vi "bool-cmd-test.vi"() -> ()   [LabVIEW 2019]
uses:
  <vilib>/Rock Robotics/WPI/ThirdParty/JAS_Junk/TrajLib/VI/BoolCmd_Recv_Internal.vi
  <vilib>/Rock Robotics/WPI/ThirdParty/JAS_Junk/TrajLib/VI/BoolCmd_Send_Internal.vi
  <vilib>/Rock Robotics/WPI/ThirdParty/JAS_Junk/TrajLib/VI/BoolCmd_ObtainQueue.vi
  <vilib>/Rock Robotics/WPI/ThirdParty/JAS_Junk/TrajLib/Trajectory_Library.lvlib
panel:
  out "Two Falling Edge":bool
  out "error out 8":errorcluster
  out "error out 7":errorcluster
  out "Two":bool
  out "One Always":bool
  out "One Edge":bool
  out "error out 6":errorcluster
  out "error out 5":errorcluster
  out "error out 4":errorcluster
  out "error out 3":errorcluster
  out "error out 2":errorcluster
  out "error out":errorcluster
  in  "milliseconds to wait 2":u32=250
  in  "milliseconds to wait":u32=250
  in  "Test 2":bool
  in  "Test 1":bool
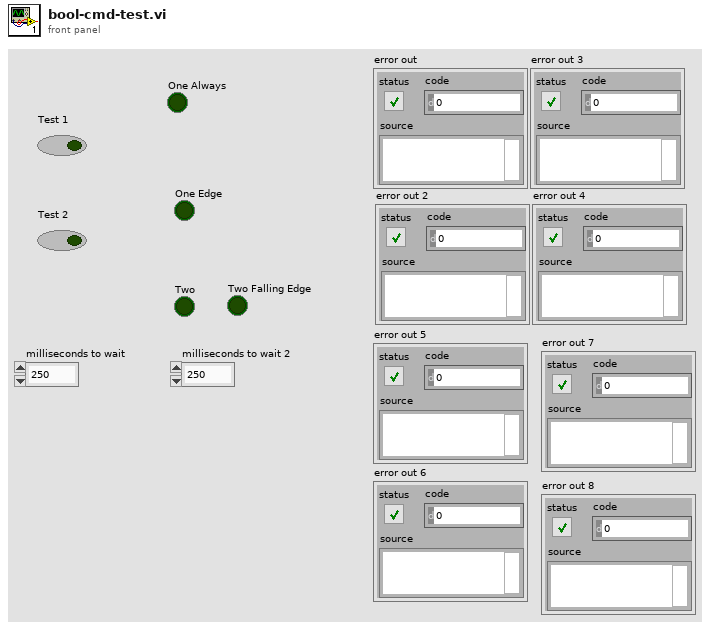
[diagram p1: front panel]
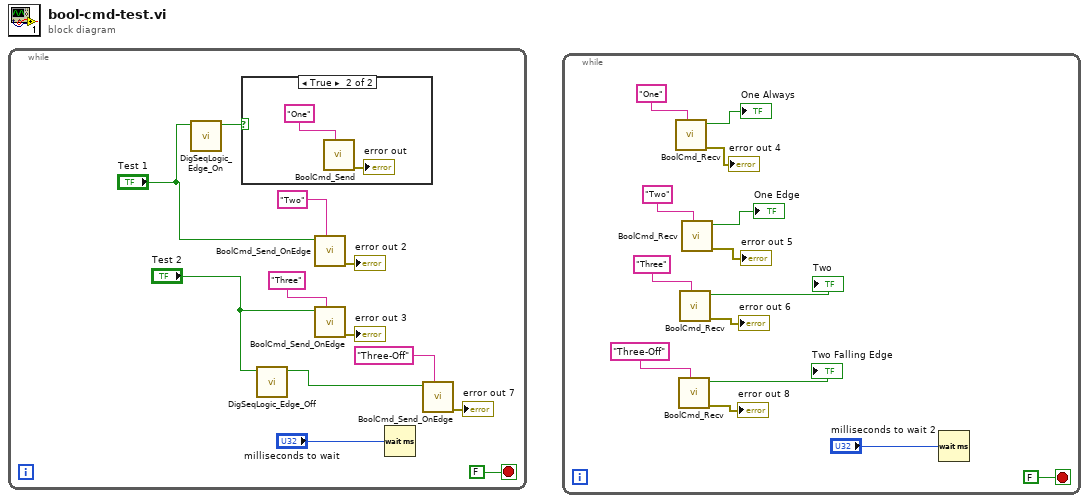
[diagram p0: block diagram]
diagram:
  n1 = while {
    stop <- FALSE stop-if-true
    n2 = call <vilib>:"DigSeqLogic_Edge_On.vi"("Input"="Test 1") -> ("On Edge"=w4:bool)  [unwired: 10 in]
    n3 = case shown="True" w4 {
      frame False {
      }
      frame True {
        n4 = call <vilib>:"BoolCmd_Send.vi"("Command Name"="One") -> ("error out"=→"error out":errorcluster)  [unwired: 10 in]
      }
    }
    n5 = call <vilib>:"DigSeqLogic_Edge_Off.vi"("Input"="Test 2") -> ("Off Edge"=w1:bool)  [unwired: 10 in]
    n6 = call <vilib>:"BoolCmd_Send_OnEdge.vi"("Command Name"="Two", "Value"="Test 1") -> ("error out"=→"error out 2":errorcluster)  [unwired: 9 in]
    n7 = call <vilib>:"BoolCmd_Send_OnEdge.vi"("Command Name"="Three", "Value"="Test 2") -> ("error out"=→"error out 3":errorcluster)  [unwired: 9 in]
    n8 = Wait (ms)(milliseconds to wait="milliseconds to wait") -> ()  [unwired: 1 out]
    n9 = call <vilib>:"BoolCmd_Send_OnEdge.vi"("Command Name"="Three-Off", "Value"=w1) -> ("error out"=→"error out 7":errorcluster)  [unwired: 9 in]
  }
  n10 = while {
    stop <- FALSE stop-if-true
    n11 = call <vilib>:"BoolCmd_Recv.vi"("Command Name"="One") -> ("error out"=→"error out 4":errorcluster, "New Request"=→"One Always":bool)  [unwired: 9 in]
    n12 = call <vilib>:"BoolCmd_Recv.vi"("Command Name"="Three-Off") -> ("error out"=→"error out 8":errorcluster, "New Request"=→"Two Falling Edge":bool)  [unwired: 9 in]
    n13 = call <vilib>:"BoolCmd_Recv.vi"("Command Name"="Three") -> ("error out"=→"error out 6":errorcluster, "New Request"=→"Two":bool)  [unwired: 9 in]
    n14 = call <vilib>:"BoolCmd_Recv.vi"("Command Name"="Two") -> ("error out"=→"error out 5":errorcluster, "New Request"=→"One Edge":bool)  [unwired: 9 in]
    n15 = Wait (ms)(milliseconds to wait="milliseconds to wait 2") -> ()  [unwired: 1 out]
  }
